vi "Create.vi"(10 "EnQr":refnum<class "Message Enqueuer.lvclass">) -> (3 "TaskEnQrValue out":refnum<class "TaskEnQrValue.lvclass">)   [LabVIEW 2020, in "Volatus.lvlib" / "TaskEnQrValue.lvclass"]
uses:
  TaskEnQrValue.lvclass
  TaskEnQrValue.lvclass/TaskEnQrValue.ctl
  <vilib>/ActorFramework/Message Enqueuer/Message Enqueuer.lvclass
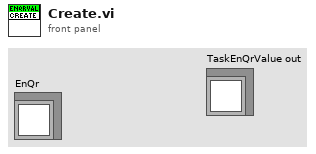
[diagram p1: front panel]
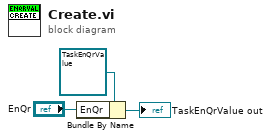
[diagram p0: block diagram]
diagram:
  n1 = Bundle By Name(cluster=refnum<class "TaskEnQrValue.lvclass"> refnum ("TaskEnQrValue in"), "EnQr"="EnQr") -> (→"TaskEnQrValue out":refnum<class "TaskEnQrValue.lvclass">)
